vi "StopMove.vi"(4 "error in":errorcluster, 5 "Stop?":bool, 6 "connection refnum in,  z":refnum<k5>, 7 "connection refnum in, xy":refnum<k5>) -> (0 "error out":errorcluster, 1 "Stop?":bool, 2 "connection refnum out z":refnum<k5>, 3 "connection refnum out xy":refnum<k5>)   [LabVIEW 2023]
doc: "Stop the motion of the instrument. Stops motors in each axis and powers off the servo motor."
uses:
  GlobalVarsNetwork.vi
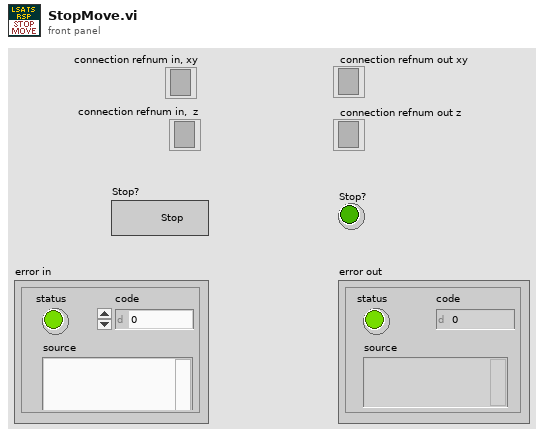
[diagram p1: front panel]
types:
  T1 = cluster{"XY_IP_ADDRESS":string, "Z_IP_ADDRESS":string, "Port":u16, "connection refnum x,y":refnum<k5>, "connection refnum z":refnum<k5>}
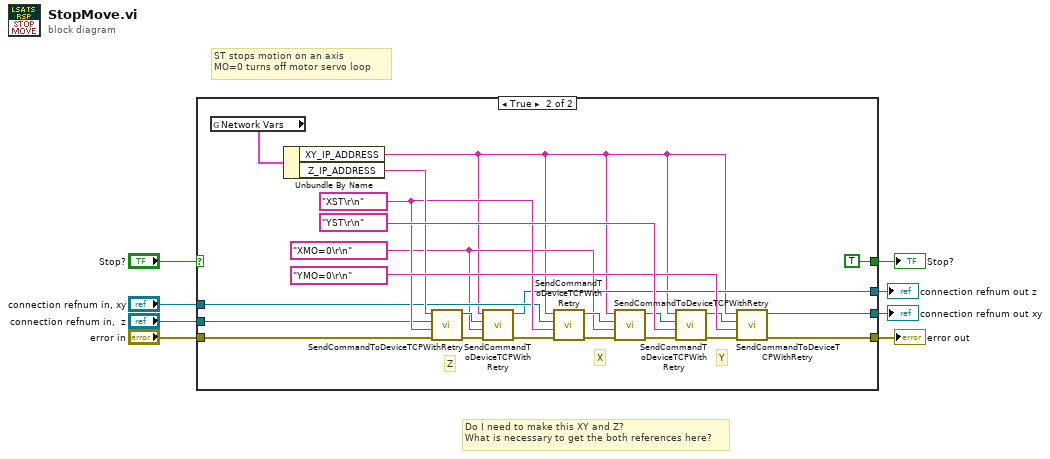
[diagram p0: block diagram]
diagram:
  # "Do I need to make this XY and Z?\nWhat is necessary to get the both references here?"
  # "ST stops motion on an axis\nMO=0 turns off motor servo loop"
  n1 = case shown="True" "Stop?" {
    selector: "Stop?" -> [w12 _]
    tunnel: "error in" -> [w11 w33]
    tunnel: [w12 TRUE] -> w6
    tunnel: [w11 w25] -> w5
    tunnel: [w9 w24] -> w3
    tunnel: [w10 w16] -> w4
    tunnel: "connection refnum in,  z" -> [w10 w20]
    tunnel: "connection refnum in, xy" -> [w9 w19]
    frame False {
    }
    frame True {
      w14 = "XMO=0\r\n"
      w26 = "XST\r\n"
      # "Y"
      # "X"
      # "Z"
      n2 = global read "GlobalVarsNetwork.vi" "Network Vars"() -> (w35:T1)
      n3 = Unbundle By Name(w35) -> ("XY_IP_ADDRESS"=w13:string, "Z_IP_ADDRESS"=w27:string)
      n4 = call "SendCommandToDeviceTCPWithRetry.vi"("error in"=w33, "str command"=w26, "connection refnum in"=w20, "IP address"=w27) -> ("error out"=w18:errorcluster, "connection refnum out"=w17:refnum<k5>)  [unwired: 4 in, 2 out]
      n5 = call "SendCommandToDeviceTCPWithRetry.vi"("error in"=w18, "str command"=w14, "connection refnum in"=w17, "IP address"=w13) -> ("error out"=w15:errorcluster, "connection refnum out"=w16:refnum<k5>)  [unwired: 4 in, 2 out]
      n6 = call "SendCommandToDeviceTCPWithRetry.vi"("error in"=w15, "str command"=w26, "connection refnum in"=w19, "IP address"=w13) -> ("error out"=w32:errorcluster, "connection refnum out"=w23:refnum<k5>)  [unwired: 4 in, 2 out]
      n7 = call "SendCommandToDeviceTCPWithRetry.vi"("error in"=w32, "str command"=w14, "connection refnum in"=w23, "IP address"=w13) -> ("error out"=w30:errorcluster, "connection refnum out"=w22:refnum<k5>)  [unwired: 4 in, 2 out]
      n8 = call "SendCommandToDeviceTCPWithRetry.vi"("error in"=w30, "str command"="YST\r\n", "connection refnum in"=w22, "IP address"=w13) -> ("error out"=w31:errorcluster, "connection refnum out"=w21:refnum<k5>)  [unwired: 4 in, 2 out]
      n9 = call "SendCommandToDeviceTCPWithRetry.vi"("error in"=w31, "str command"="YMO=0\r\n", "connection refnum in"=w21, "IP address"=w13) -> ("error out"=w25:errorcluster, "connection refnum out"=w24:refnum<k5>)  [unwired: 4 in, 2 out]
    }
  }
  "Stop?" <- w6
  "error out" <- w5
  "connection refnum out z" <- w4
  "connection refnum out xy" <- w3
